vi "verify_new_color_channel.vi"(8 "error in (no error)":errorcluster, 9 "channel colours new":T1[](array[typedef])=[enum."red", enum."green", enum."blue", enum."red"], 10 "channel colours old":T1[](array[typedef])=[enum."red", enum."green", enum."blue", enum."red"]) -> (0 "error out":errorcluster, 2 "channel colours out":T1[](array[typedef])=[enum."red", enum."green", enum."blue", enum."red"])   [LabVIEW 2010, in "DisplayDL090216.lvclass"]
uses:
  DisplayDL090216.lvclass
  common/enumerations/channel_display_colour_enum.ctl
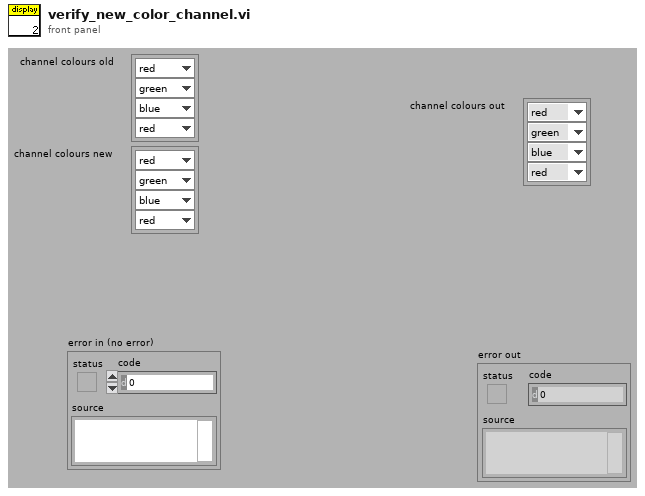
[diagram p1: front panel]
types:
  T1 = typedef "channel_display_colour_enum.ctl" = enum16{"none", "red", "green", "blue", "grey scale", "custom"}
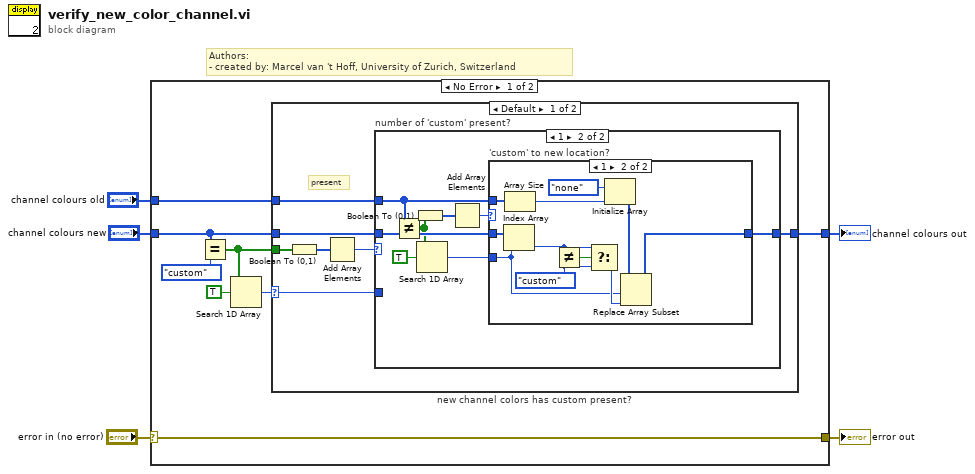
[diagram p0: block diagram]
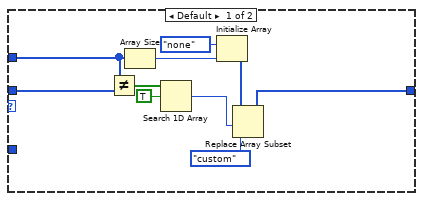
[diagram p2: hidden frame]
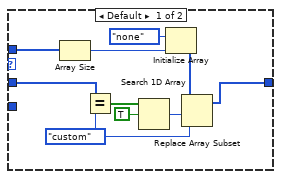
[diagram p3: hidden frame]
diagram:
  # "Authors: \n- created by: Marcel van 't Hoff, University of Zurich, Switzerland"
  n1 = case shown="No Error" "error in (no error)" {
    selector: "error in (no error)" -> [w13 w61]
    tunnel: [w13 w61] -> w4
    tunnel: "channel colours old" -> [w9 _]
    tunnel: "channel colours new" -> [w10 _]
    tunnel: [w11 _] -> w1
    frame No Error {
      n2 = Equal?(x=w10, y=channel_display_colour_enum."custom" ("channel x")) -> (x = y?=w6:bool[])
      n3 = Search 1D Array(1D array=w6, element=TRUE) -> (index of element=w7:i32)  [unwired: 1 in]
      n4 = case "new channel colors has custom present?" shown="Default" w7 {
        selector: w7 -> [w15 _]
        tunnel: [w14 w60] -> w11
        tunnel: w10 -> [w16 w60]
        tunnel: w9 -> [w20 _]
        tunnel: w6 -> [w19 _]
        frame Default {
          # "present"
          n5 = Boolean To (0,1)(Boolean=w19) -> (0, 1=w18:i16[])
          n6 = Add Array Elements(numeric array=w18) -> (sum=w17:i16)
          n7 = case "number of 'custom' present?" shown="1" w17 {
            tunnel: w20 -> [w23 w38]
            tunnel: w16 -> [w30 w35]
            tunnel: w15 -> [_ _]
            tunnel: [w21 w34] -> w14
            frame Default {
              n8 = Not Equal?(x=w23, y=w30) -> (x != y?=w28:bool[])
              n9 = Array Size(array=w23) -> (size(s)=w27:i32)
              n10 = Search 1D Array(1D array=w28, element=TRUE) -> (index of element=w22:i32)  [unwired: 1 in]
              n11 = Initialize Array(channel_display_colour_enum."none" ("channel x"), w27) -> (w25:T1[])
              n12 = Replace Array Subset(array=w25, new element=channel_display_colour_enum."custom" ("channel x"), index=w22) -> (w21:T1[])
            }
            frame 1 {
              n13 = Not Equal?(x=w38, y=w35) -> (x != y?=w32:bool[])
              n14 = Boolean To (0,1)(Boolean=w32) -> (0, 1=w33:i16[])
              n15 = Search 1D Array(1D array=w32, element=TRUE) -> (index of element=w36:i32)  [unwired: 1 in]
              n16 = Add Array Elements(numeric array=w33) -> (sum=w31:i16)
              n17 = case "'custom' to new location?" shown="1" w31 {
                tunnel: w38 -> [w43 w56]
                tunnel: w36 -> [_ w51]
                tunnel: w35 -> [w48 w50]
                tunnel: [w39 w49] -> w34
                frame Default {
                  w40 = channel_display_colour_enum."custom" ("channel x")
                  n18 = Array Size(array=w43) -> (size(s)=w45:i32)
                  n19 = Equal?(x=w48, y=w40) -> (x = y?=w46:bool[])
                  n20 = Search 1D Array(1D array=w46, element=TRUE) -> (index of element=w41:i32)  [unwired: 1 in]
                  n21 = Initialize Array(channel_display_colour_enum."none" ("channel x"), w45) -> (w42:T1[])
                  n22 = Replace Array Subset(array=w42, new element=w40, index=w41) -> (w39:T1[])
                }
                frame 1 {
                  w53 = channel_display_colour_enum."custom" ("channel x")
                  n23 = Index Array(array=w50, index=w51) -> (element=w54:T1)
                  n24 = Array Size(array=w56) -> (size(s)=w59:i32)
                  n25 = Not Equal?(x=w54, y=w53) -> (x != y?=w55:bool)
                  n26 = Select(t=w54, s=w55, f=w53) -> (s? t:f=w52:T1)
                  n27 = Initialize Array(channel_display_colour_enum."none" ("channel x"), w59) -> (w57:T1[])
                  n28 = Replace Array Subset(array=w57, new element=w52, index=w51) -> (w49:T1[])
                }
              }
            }
          }
        }
        frame -1 {
          # "non present"
        }
      }
    }
    frame Error {
    }
  }
  "error out" <- w4
  "channel colours out" <- w1
